vi "Build Game Board.vi"(8 "error in (no error)":errorcluster, 9 "Active Pixels":cluster{"Column":u8, "Row":u8, "Color":u32}[](array[cluster]), 10 "Board To Draw":u32[][](array[numeric]), 11 "Screen Interface in":refnum<class "Screen Interface.lvclass">) -> (0 "error out":errorcluster, 3 "Screen Interface out":refnum<class "Screen Interface.lvclass">)   [LabVIEW 2017, in "Screen Interface.lvlib" / "Screen Interface.lvclass"]
uses:
  Screen Interface.lvclass
  Screen Interface.lvclass/Screen Interface.ctl
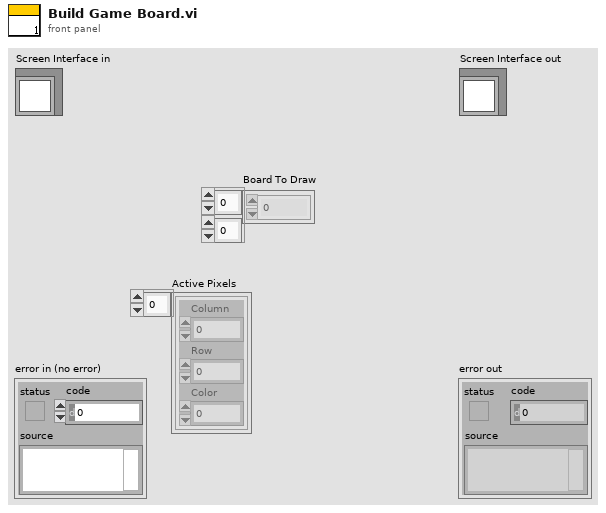
[diagram p1: front panel]
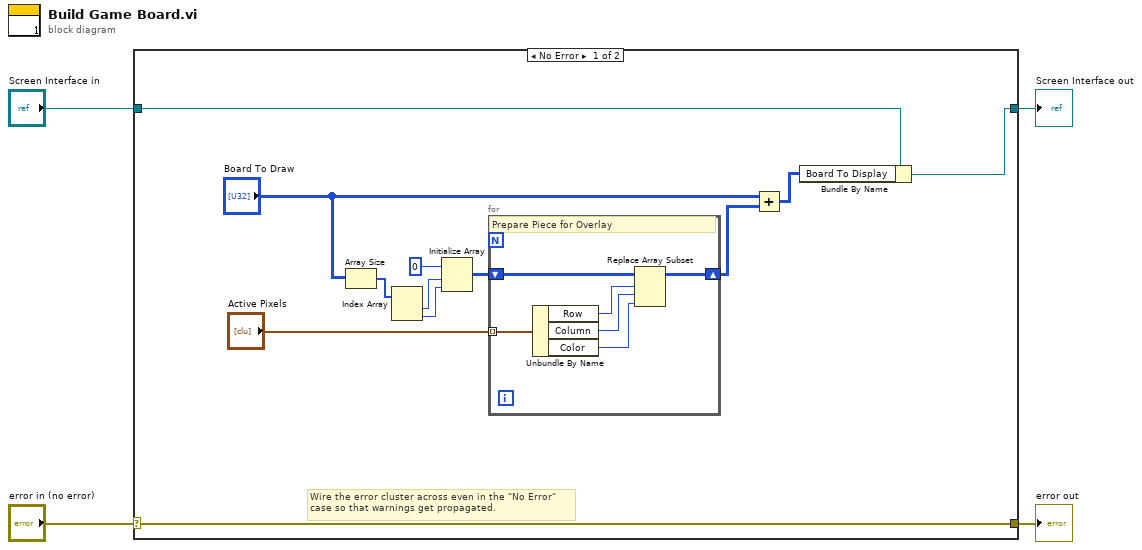
[diagram p0: block diagram]
diagram:
  n1 = case shown="No Error" "error in (no error)" {
    selector: "error in (no error)" -> [w16 w24]
    tunnel: [w16 w24] -> w3
    tunnel: [w5 w23] -> w1
    tunnel: "Screen Interface in" -> [w7 w23]
    frame No Error {
      # "Wire the error cluster across even in the \"No Error\"\ncase so that warnings get propagated."
      n2 = Array Size(array="Board To Draw") -> (size(s)=w13:i32[])
      n3 = Index Array(array=w13) -> (element #1=w12:i32, element #2=w11:i32)  [unwired: 2 in]
      n4 = Initialize Array(u32 0, w12, w11) -> (w14:u32[][])
      n5 = for {
        shift-right: [w19] -> w10
        shift-left: w14 -> [w22]
        tunnel: "Active Pixels" -> [w18] mode=indexing
        # "Prepare Piece for Overlay"
        n6 = Unbundle By Name(w18) -> ("Row"=w21:u8, "Column"=w20:u8, "Color"=w17:u32)
        n7 = Replace Array Subset(array=w22, new element=w17, index (row)=w21, index (col)=w20) -> (w19:u32[][])
      }
      n8 = Add(x="Board To Draw", y=w10) -> (x+y=w6:u32[][])
      n9 = Bundle By Name(cluster=w7, "Board To Display"=w6) -> (w5:refnum<class "Screen Interface.lvclass">)
    }
    frame Error {
    }
  }
  "error out" <- w3
  "Screen Interface out" <- w1
